vi "Stopped.vi"(6 "Teller":refnum<class "Teller.lvclass">, 9 "Error":errorcluster, 10 "Actor":refnum<class "Actor.lvclass">, 11 "Core Actor in":refnum<class "Core Actor.lvclass">) -> (0 "Error out":errorcluster, 3 "Core Actor out":refnum<class "Core Actor.lvclass">)   [LabVIEW 2025, in "jettl.lvlib" / "Core Actor.lvlib" / "Core Actor.lvclass"]
uses:
  Core Actor.lvclass
  C:/git/jettl/src/jettl/jettl/Actor/Actor.lvclass
  Actor/Actor.lvclass
  Teller/Teller/Teller.lvclass
  Core Actor.lvclass/Core Actor.ctl
  Stop Msg/Call.vi
  Attributes/Attributes/Attributes.lvclass
  C:/git/jettl/src/jettl/jettl/Core Actor/Core Actor/Core Actor.lvclass
  C:/git/jettl/src/jettl/jettl/Stop Msg/Stop/Stop.lvclass
  C:/git/jettl/src/jettl/jettl/Stopped Msg/Stopped/Stopped.lvclass
  Stop Msg/Stop Msg.lvlib
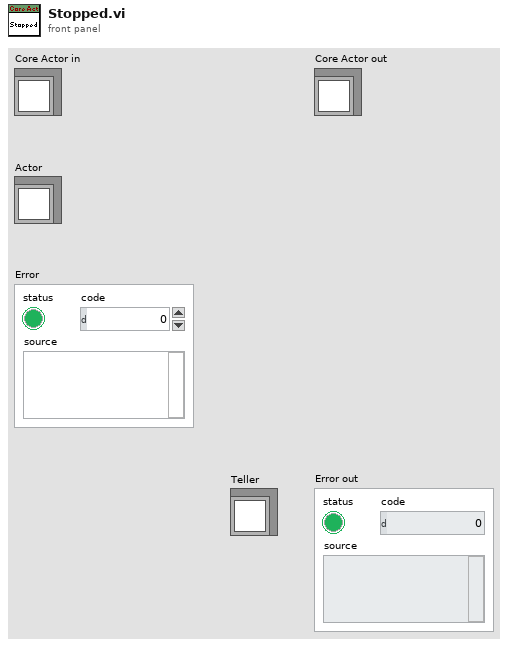
[diagram p1: front panel]
types:
  T1 = typedef "jettl.lvlib/Relation.ctl" = enum16{"Self", "Parent", "Child"}
  T2 = typedef "jettl.lvlib/Core Actor.lvlib/Core Actor.lvclass/Child Attributes Map.ctl" = map{string, refnum<class "Attributes.lvclass">}
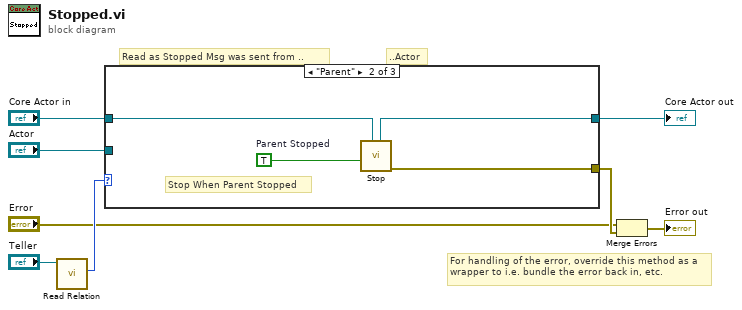
[diagram p0: block diagram]
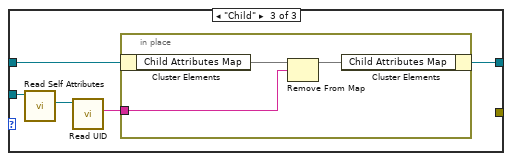
[diagram p3: hidden frame]
diagram:
  # "For handling of the error, override this method as a wrapper to i.e. bundle the error back in, etc."
  # "..Actor"
  # "Read as Stopped Msg was sent from .."
  n1 = call-dynamic "Read Relation.vi"("Teller in"="Teller") -> ("Relation"=w4:T1)  [unwired: 10 in]
  n2 = case shown="\"Parent\"" w4 {
    tunnel: "Core Actor in" -> [w9 w11 w17]
    tunnel: [w9 w13 w14] -> w8
    tunnel: "Actor" -> [_ _ w18]
    tunnel: [_ w12 _] -> w2
    frame "Self" {
      # "Case will not fundamentally execute"
    }
    frame "Parent" {
      w10 = TRUE  # Parent Stopped
      # "Stop When Parent Stopped"
      n3 = call-poly "Stop.vi"("Actor in"=w11, "Parent Stopped"=w10) -> ("Error out"=w12:errorcluster, "Actor out"=w13:refnum<class "Core Actor.lvclass">)  [unwired: 8 in]
    }
    frame "Child" {
      n4 = call-dynamic "Read Self Attributes.vi"("Actor in"=w18) -> ("Self Attributes"=w16:refnum<class "Attributes.lvclass">)  [unwired: 10 in]
      n5 = call-dynamic "Read UID.vi"("Attributes in"=w16) -> ("UID"=w15:string)  [unwired: 10 in]
      n6 = in-place {
        in-place-border: w15 -> [w19]
        n7 = in-place-cluster #1(w17) -> ("Child Attributes Map"=w21:T2)
        n8 = Remove From Map(10:w19, 11:w21) -> (3:w20:T2)  [unwired: 2 out]
        n9 = in-place-cluster #1("Child Attributes Map"=w20) -> (w14:refnum<class "Core Actor.lvclass">)
      }
    }
  }
  "Core Actor out" <- w8
  n10 = Merge Errors("Error", w2) -> (→"Error out":errorcluster)
